vi "直通基准单次测试.vi"(8 "error in":errorcluster, 9 "out":i32=1, 11 "in":i32=2) -> (0 "error out":errorcluster)   [LabVIEW 2015]
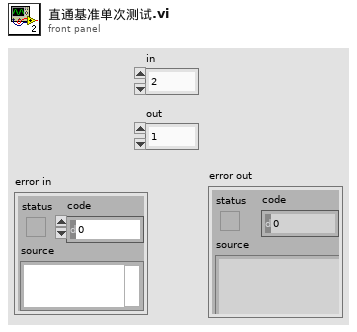
[diagram p1: front panel]
types:
  T1 = typedef "直通基准state.ctl" = enum16{"Idle", "开始消息", "切换开关", "网分测量", "数据库操作", "结束消息"}
  T2 = cluster{"Freq":dbl[], "S11":dbl[], "S12":dbl[], "S21":dbl[], "S22":dbl[]}
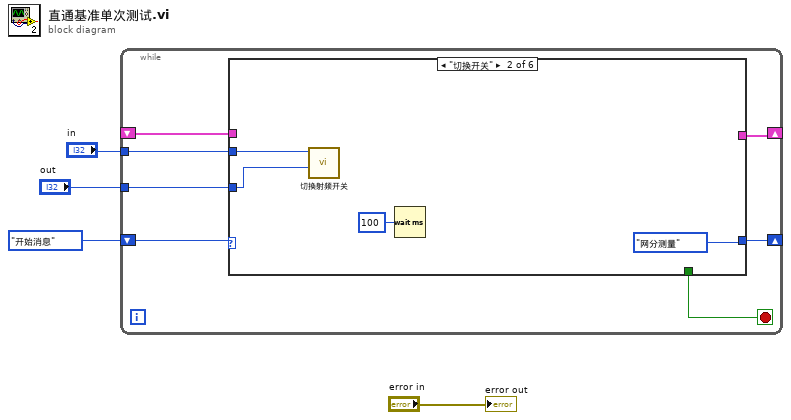
[diagram p0: block diagram]
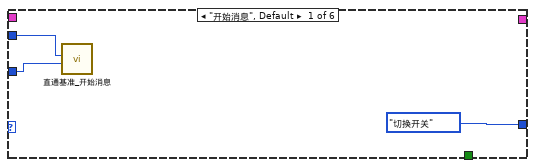
[diagram p2: hidden frame]
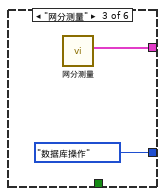
[diagram p3: hidden frame]
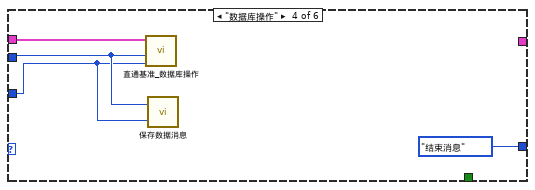
[diagram p4: hidden frame]
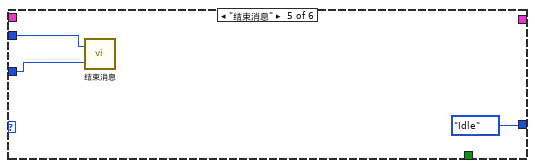
[diagram p5: hidden frame]
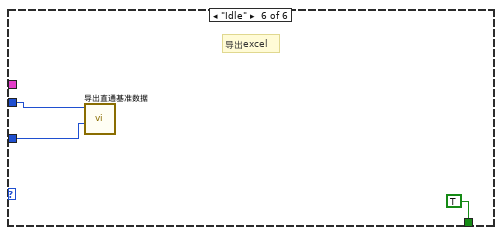
[diagram p6: hidden frame]
diagram:
  n1 = while {
    tunnel: "in" -> [w11]
    tunnel: "out" -> [w10]
    shift-right: [w8] -> _
    shift-left: 直通基准state."开始消息" ("直通基准State") -> [w9]
    shift-right: [w7] -> _
    shift-left: _ -> [w6]
    stop <- w5 stop-if-true
    n2 = case shown="\"切换开关\"" w9 {
      tunnel: w11 -> [w14 w16 _ w22 w26 w29]
      tunnel: w10 -> [w13 w15 _ w21 w25 w28]
      tunnel: [直通基准state."切换开关" ("直通基准State") 直通基准state."网分测量" ("直通基准State") 直通基准state."数据库操作" ("直通基准State") 直通基准state."结束消息" ("直通基准State") 直通基准state."Idle" ("直通基准State") _] -> w8
      tunnel: [_ _ w20 _ _ _] -> w7
      tunnel: w6 -> [_ _ _ w24 _ _]
      tunnel: [_ _ _ _ _ TRUE] -> w5
      frame "开始消息", Default {
        n3 = call "直通基准_开始消息.vi"("COM"=w13, "A"=w14) -> ()  [unwired: 10 in]
      }
      frame "切换开关" {
        n4 = call "切换射频开关.vi"("COM"=w15, "A"=w16) -> ()  [unwired: 7 in, 3 out]
        n5 = Wait (ms)(milliseconds to wait=u32 100) -> ()  [unwired: 1 out]
      }
      frame "网分测量" {
        n6 = call "网分测量.vi"() -> ("Freq&S"=w20:T2)  [unwired: 11 in]
      }
      frame "数据库操作" {
        n7 = call "直通基准_数据库操作.vi"("出口"=w21, "进口"=w22, "Freq&S"=w24) -> ()  [unwired: 9 in]
        n8 = call "保存数据消息.vi"("COM"=w21, "A"=w22) -> ()  [unwired: 1 in]
      }
      frame "结束消息" {
        n9 = call "结束消息.vi"("COM"=w25, "A"=w26) -> ()  [unwired: 1 in]
      }
      frame "Idle" {
        # "导出excel"
        n10 = call "导出直通基准数据.vi"("OUT"=w28, "IN"=w29) -> ()  [unwired: 9 in, 1 out]
      }
    }
  }
  "error out" <- "error in"
